vi "Edgertronic-:get_storage_dir copy.vi"(5 "Setup":T2={"URL"="130.64.16.195", "remote port"=80, "mode (standard)"=enum."Standard"}) -> (0 "error out":errorcluster, 1 "Storage Dir:":T1={"Storage Dir"="20140911165611", "Connection Information:"=""}, 2 "data out":string="HTTP/1.0 200 OK\r\nContent-Type: text/html; charset=utf-8\r\nContent-Length: 313\r\nConnection: close\r\nDate: Tue, 16 Jun 2015 13:54:12 GMT\r\nServer: lighttpd/1.4.11 (edgertonic slow motion camera)\r\n\r\n{\"build_date\": \"20150112\", \"sw_build_date\": \"20140911165611\", \"fpga_initialized\": 1, \"hardware_revision\": 6, \"model_number\": 1, \"home_dir\": \"/home/root/ss-web\", \"ir_filter\": 1, \"mac_addr\": \"00:1B:C5:09:61:4D\", \"serial_console_enabled\": false, \"serial_number\": 333, \"fpga_version\": 70, \"hardware_configuration\": 1}")   [LabVIEW 2012]
doc: "This VI returns the mount point of the active storage device."
panel:
  in  "GET Cmd":string="/get_storage_dir"
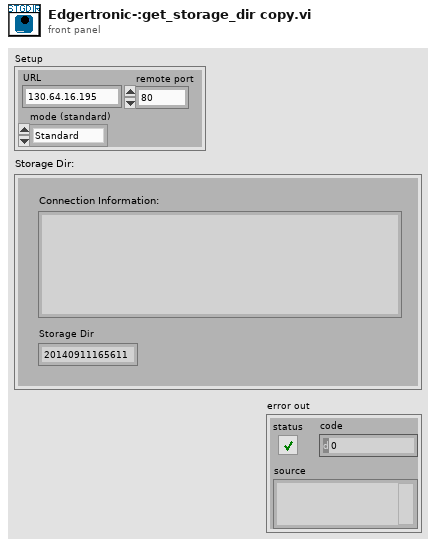
[diagram p1: front panel]
types:
  T1 = cluster{"Storage Dir":string, "Connection Information:":string}
  T2 = cluster{"URL":string, "remote port":u16, "mode (standard)":enum16{"Standard", "Buffered", "CRLF", "Immediate"}}
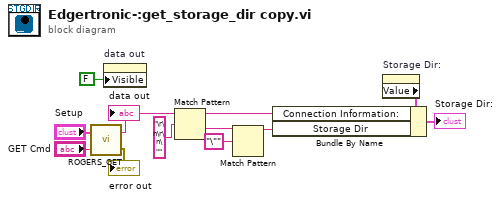
[diagram p0: block diagram]
diagram:
  n1 = call <userlib>:"ROGERS_GET.vi"("GET Cmd"="GET Cmd", "Setup"="Setup") -> ("error out"=→"error out":errorcluster, "data out"=w9:string)
  "data out" <- w9
  n2 = property on="data out" class="Str"("Visible"=FALSE) -> ()  [unwired: 2 in, 2 out]
  n3 = Match Pattern(string=w9, regular expression="\r\n\r\n\"") -> (before substring=w7:string, after substring=w4:string)  [unwired: 1 in, 2 out]
  n4 = Match Pattern(string=w4, regular expression="\"") -> (before substring=w3:string)  [unwired: 1 in, 3 out]
  n5 = property on="Storage Dir:" class="Clust (strict)"() -> ("Value"=w1:T1)  [unwired: 2 in, 2 out]
  n6 = Bundle By Name(cluster=w1, "Connection Information:"=w7, "Storage Dir"=w3) -> (→"Storage Dir:":T1)
